vi "example_03_info.vi"() -> ()   [LabVIEW 2015, in "lv-dropbox.lvlib" / "v2.lvlib"]
uses:
  v2.lvlib
  public/advanced/list_folder-basic.vi
panel:
  out "used":dbl
  out "allocated":dbl
  out "remaining":dbl
  out "error out":errorcluster
  out "path []":string[](array[string])
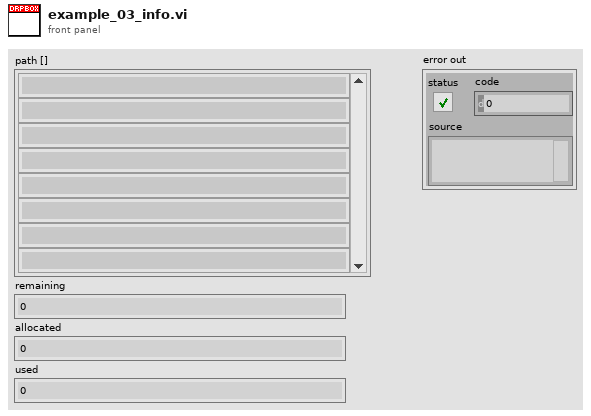
[diagram p1: front panel]
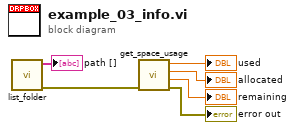
[diagram p0: block diagram]
diagram:
  n1 = call-poly "list_folder.vi"() -> ("error out"=w6:errorcluster, "path []"=→"path []":string[])  [unwired: 9 in, 1 out]
  n2 = call "get_space_usage.vi"("error in (no error)"=w6) -> ("error out"=→"error out":errorcluster, "remaining"=→"remaining":dbl, "allocated"=→"allocated":dbl, "used"=→"used":dbl)  [unwired: 7 in]
